vi "HSDIO_6541_Load_Wfm_Script.vi"(8 "error  in":errorcluster caption="error in", 9 "TIMING Inputs":T2={"Number of Acquisitions "=1, "Number of Accumulations"=1, "Table of Waveforms"=[], "Script Text"=""} {"Number of Accumulations" min=0 max=50 step=1; "Number of Acquisitions" min=1 max=10 step=1}, 10 "SOFTWARE Inputs":T1={"Application Directory"=path "D:/S.O.F.T.S/LABVIEW/PIL", "Software Version"="1.0.0", "Data Path"=path "D:/PIRENEA/DATA", "XML Path"=path "D:/PIRENEA/DATA", "XML File Filter"="*.xml", "XML Saved Path"=path "D:/PIRENEA/DATA/SAVED", "Excit Scripts Path"=path "D:/PIRENEA/TECHNICAL/EXCIT_SCRIPTS", "Excit Scripts File Filter"="*.txt", "Excit Waveforms Path"=path "D:/PIRENEA/TECHNICAL/EXCIT_WFMS", "Excit Waveforms File Filter"="*.bin", "Timing Scripts Path"=path "D:/PIRENEA/TECHNICAL/TIMING_SCRIPTS", "Timing Scripts File Filter"="*.txt", "Timing Waveforms Path"=path "D:/PIRENEA/TECHNICAL/TIMING_WFMS", "Timing Waveforms File Filter"="*.bin", "Trapping Waveforms Path"=path "D:/PIRENEA/TECHNICAL/TRAPPING_WFMS", "Trapping Waveforms File Filter"="*.bin"}, 11 "instrument handle in":refnum<k15>="Sequencer") -> (0 "error out":errorcluster, 1 "Script text":string, 2 "FIFO used":i64, 3 "instrument handle out":refnum<k15>)   [LabVIEW 2020]
doc: "This VI demonstrates how to load dynamic waveforms into the board.\n\n1. The waveform binary files are read one by one from the waveform folder.\n2. The data are converted to U32 format and loaded into the on-board memory.\n\nThis VI returns the max memory size of the board, the memory used after loading, and a list of the waveforms loaded. No check of memory overflow is done."
uses:
  controls/TIMING_Inputs.ctl
  controls/SOFTWARE_Inputs.ctl
  <instrlib>/niHSDIO/niHSDIO.llb/niHSDIO Write Named Waveform (1D U32).vi
panel:
  out "FIFO max size":i32
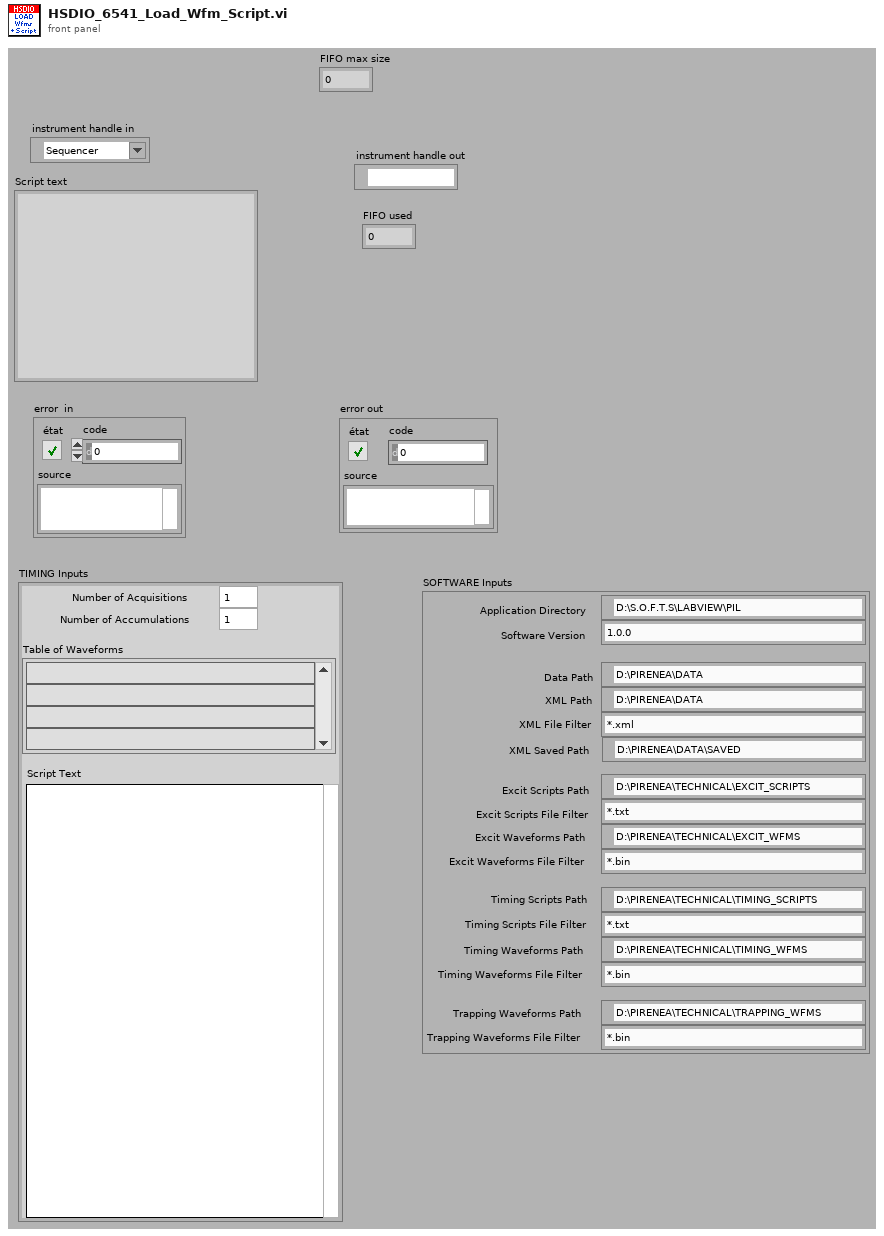
[diagram p1: front panel]
types:
  T1 = typedef "SOFTWARE_Inputs.ctl" = cluster{"Application Directory":path, "Software Version":string, "Data Path":path, "XML Path":path, "XML File Filter":string, "XML Saved Path":path, "Excit Scripts Path":path, "Excit Scripts File Filter":string, "Excit Waveforms Path":path, "Excit Waveforms File Filter":string, "Timing Scripts Path":path, "Timing Scripts File Filter":string, "Timing Waveforms Path":path, "Timing Waveforms File Filter":string, "Trapping Waveforms Path":path, "Trapping Waveforms File Filter":string}
  T2 = typedef "TIMING_Inputs.ctl" = cluster{"Number of Acquisitions ":i16, "Number of Accumulations":i16, "Table of Waveforms":string[], "Script Text":string}
  T3 = enum16{"big-endian, network order", "native, host order", "little-endian"}
  T4 = enum16{"open", "replace", "create", "open or create", "replace or create", "replace or create with confirmation"}
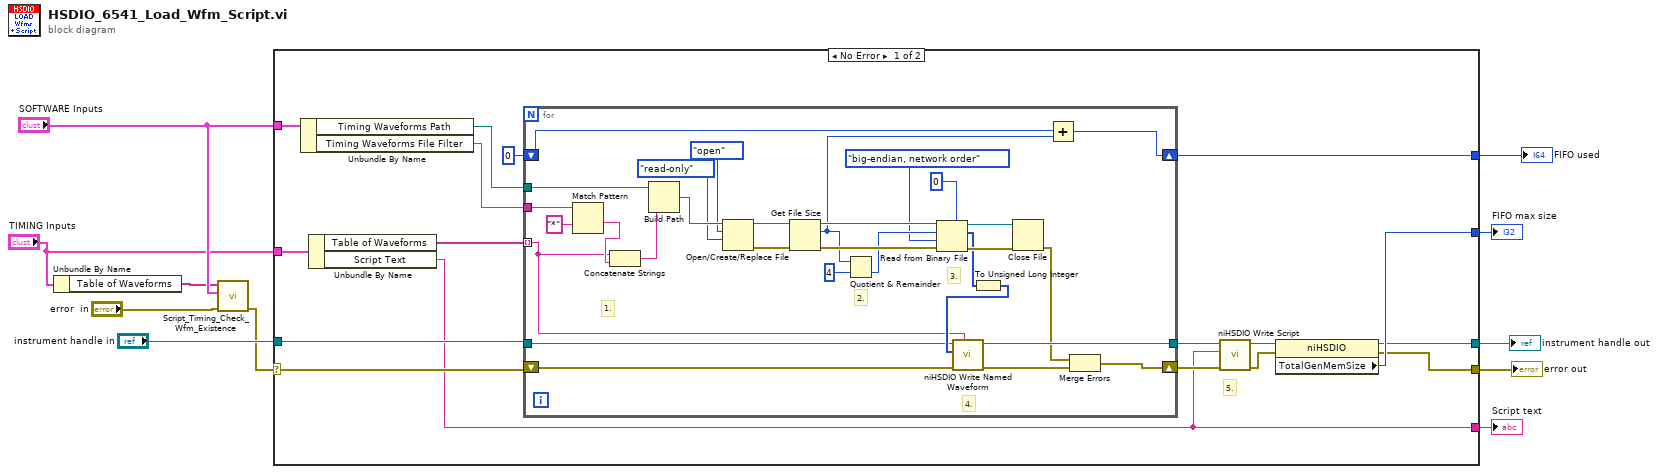
[diagram p0: block diagram]
diagram:
  n1 = Unbundle By Name("TIMING Inputs") -> ("Table of Waveforms"=w1:string[])
  n2 = call "Script_Timing_Check_Wfm_Existence.vi"("error  in"="error  in", "SOFTWARE Inputs"="SOFTWARE Inputs", "Table of Waveforms"=w1) -> ("error out"=w3:errorcluster)  [unwired: 8 in]
  n3 = case shown="No Error" w3 {
    selector: w3 -> [w27 w59]
    tunnel: [w13 w59] -> w11
    tunnel: [w14 w60] -> w10
    tunnel: "instrument handle in" -> [w28 w60]
    tunnel: "SOFTWARE Inputs" -> [w22 _]
    tunnel: "TIMING Inputs" -> [w19 _]
    tunnel: [w16 _] -> w8
    tunnel: [w15 _] -> w7
    tunnel: [w12 _] -> w6
    frame No Error {
      # "5."
      n4 = Unbundle By Name(w22) -> ("Timing Waveforms Path"=w21:path, "Timing Waveforms File Filter"=w20:string)
      n5 = Unbundle By Name(w19) -> ("Table of Waveforms"=w18:string[], "Script Text"=w12:string)
      n6 = for {
        shift-right: [w35] -> w24
        shift-left: w27 -> [w43]
        tunnel: w28 -> [w42]
        tunnel: [w41] -> w25
        shift-right: [w39] -> w16
        shift-left: i64 0 -> [w38]
        tunnel: w18 -> [w30] mode=indexing
        tunnel: w21 -> [w34]
        tunnel: w20 -> [w33]
        # "4."
        # "3."
        # "2."
        # "1."
        n7 = Match Pattern(string=w33, regular expression="*" ("expression régulière")) -> (after substring=w31:string)  [unwired: 1 in, 3 out]
        n8 = Concatenate Strings(w30, w31) -> (w29:string)
        n9 = Build Path(base path=w34, name or relative path=w29) -> (appended path=w56:path)
        n10 = Open/Create/Replace File(file path (use dialog)=w56, operation (0:open)=T4."open", access (0:read/write)=enum16{"read/write", "read-only", "write-only"}."read-only") -> (refnum out=w58:refnum<file>, error out=w57:errorcluster)  [unwired: 3 in, 1 out]
        n11 = Get File Size(file=w58, error in=w57) -> (refnum out=w52:refnum<file>, size (in bytes)=w40:i64, 0:w50:errorcluster)
        n12 = Quotient & Remainder(x=w40, y=i64 4 ("type size (bytes)")) -> (floor(x/y)=w48:i64)  [unwired: 1 out]
        n13 = Read from Binary File(5:u32 0 ("data type"), 8:w50, 9:T3."big-endian, network order" ("ordre des octets (0 : big-Endian, network order)"), 10:w48, 11:w52) -> (0:w49:errorcluster, 2:w45:u32[], 3:w51:refnum<file>)  [unwired: 1 in, 1 out]
        n14 = To Unsigned Long Integer(number=w45) -> (unsigned 32bit integer=w47:u32[])
        n15 = call-poly <instrlib>:"niHSDIO Write Named Waveform.vi"("waveform name (default:\"\")"=w30, "error in (no error)"=w43, "data"=w47, "instrument handle"=w42) -> ("error out"=w36:errorcluster, "instrument handle out"=w41:refnum<k15>)  [unwired: 6 in]
        n16 = Close File(refnum=w51, error in=w49) -> (error out=w37:errorcluster)  [unwired: 1 out]
        n17 = Add(x=w38, y=w40) -> (x+y=w39:i64)
        n18 = Merge Errors(w37, w36) -> (w35:errorcluster)
      }
      n19 = call <instrlib>:"niHSDIO Write Script.vi"("error in (no error)"=w24, "script"=w12, "instrument handle"=w25) -> ("error out"=w23:errorcluster, "instrument handle out"=w17:refnum<k15>)  [unwired: 7 in]
      n20 = property on="Property Node" class="niHSDIO"(reference=w17, error in=w23) -> (reference out=w14:refnum<k15>, error out=w13:errorcluster, "TotalGenMemSize"=w15:i32)
    }
    frame Error {
    }
  }
  "error out" <- w11
  "instrument handle out" <- w10
  "FIFO used" <- w8
  "FIFO max size" <- w7
  "Script text" <- w6
